vi "getDebuggingFlag.vi"(8 "error in (no error)":errorcluster, 11 "HWController.lvclass in":refnum<class "HWController.lvclass">) -> (0 "error out":errorcluster, 2 "debuggingFlag":bool, 3 "HWController.lvclass out":refnum<class "HWController.lvclass">)   [LabVIEW 2011, in "Hardware.lvlib" / "HWControllers.lvlib" / "HWController.lvclass"]
uses:
  HWController.lvclass
  HWController.lvclass/HWController.ctl
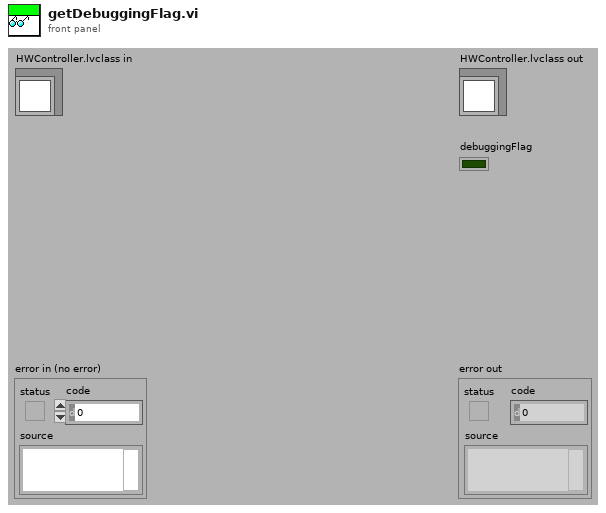
[diagram p1: front panel]
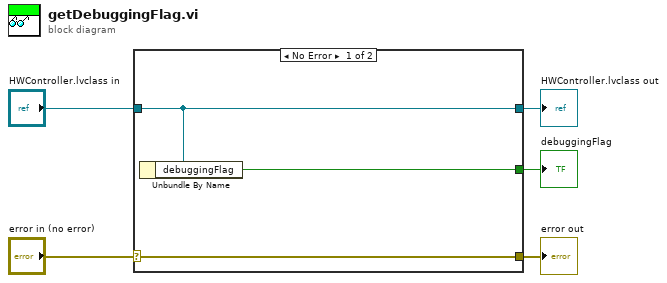
[diagram p0: block diagram]
diagram:
  n1 = case shown="No Error" "error in (no error)" {
    selector: "error in (no error)" -> [w8 w9]
    tunnel: [w8 w9] -> w4
    tunnel: [w7 w10] -> w2
    tunnel: "HWController.lvclass in" -> [w7 w10]
    tunnel: [w6 _] -> w1
    frame No Error {
      n2 = Unbundle By Name(w7) -> ("debuggingFlag"=w6:bool)
    }
    frame Error {
    }
  }
  "error out" <- w4
  "HWController.lvclass out" <- w2
  "debuggingFlag" <- w1
